vi "Set - Scalar - Real.vi"(8 "error in":errorcluster, 9 "value":dbl, 10 "variable name":string, 11 "pipe in":T1) -> (0 "error out":errorcluster, 3 "pipe out":T1)   [LabVIEW 2013, in "GOLPI library.lvlib"]
uses:
  GOLPI library.lvlib
  LV Process.lvlibp/Pipe Handle.ctl
  Globals.vi
  LV Process.lvlibp
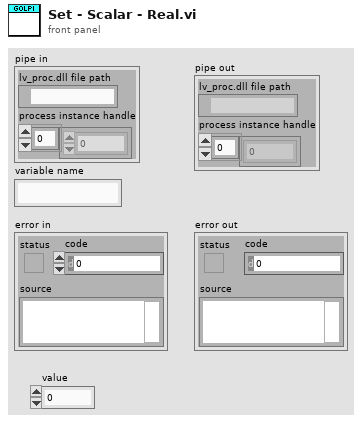
[diagram p1: front panel]
types:
  T1 = typedef "LV Process.lvlibp/Pipe Handle.ctl" = cluster{"lv_proc.dll file path":path, "process instance handle":u32[]}
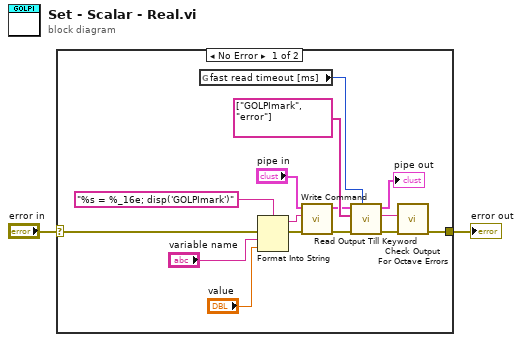
[diagram p0: block diagram]
diagram:
  n1 = case shown="No Error" "error in" {
    selector: "error in" -> [w14 w18]
    tunnel: [w3 w18] -> w2
    frame No Error {
      n2 = global read "Globals.vi" "fast read timeout [ms]"() -> (w5:u32)
      n3 = Format Into String(format string="%s = %_16e; disp('GOLPImark')", error in=w14, "variable name", "value") -> (resulting string=w11:string, error out=w13:errorcluster)  [unwired: 1 in]
      n4 = call "Write Command.vi"("error in"=w13, "command"=w11, "pipe in"="pipe in") -> ("error out"=w10:errorcluster, "pipe out"=w7:T1)  [unwired: 7 in]
      n5 = call "Read Output Till Keyword.vi"("timeout [ms]"=w5, "error in"=w10, "keywords"=string[] ["GOLPImark", "error"], "pipe in"=w7) -> ("error out"=w9:errorcluster, "read buffer"=w6:string, "pipe out"=→"pipe out":T1)  [unwired: 4 in, 1 out]
      n6 = call "Check Output For Octave Errors.vi"("error in"=w9, "read buffer"=w6) -> ("error out"=w3:errorcluster)  [unwired: 9 in]
    }
    frame Error {
    }
  }
  "error out" <- w2
